vi "数据查询_仪器数据_古田户外.vi"() -> ()   [LabVIEW 2016]
uses:
  <vilib>/Utility/miscctls.llb/LVRowAndColumnUnsignedTypeDef.ctl
  <vilib>/Utility/miscctls.llb/LVPointTypeDef.ctl
panel:
  in  "工作模式":string(combo)="全部数据"
  in  "查询":bool
  in  "结束日期":string="2020/01/01"
  in  "起始日期":string="2010/01/01"
  in  "组合框":string(combo)
  out "数据表":string[][](table)
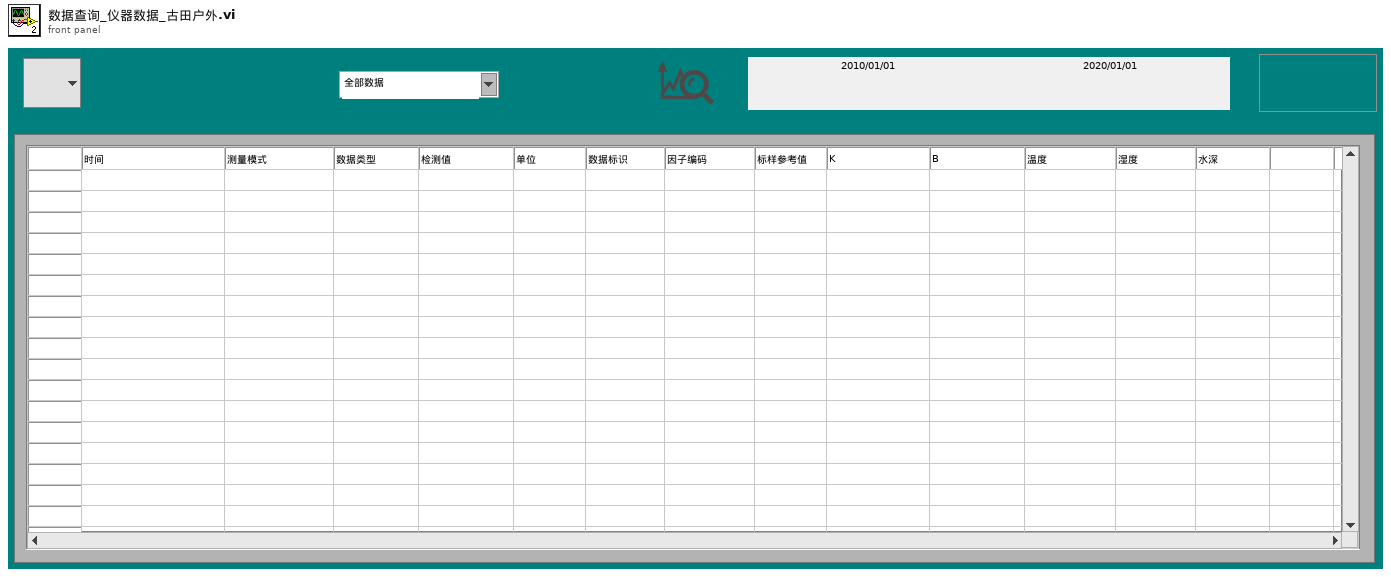
[diagram p1: front panel]
types:
  T1 = typedef "LVRowAndColumnUnsignedTypeDef.ctl" = cluster{"Row":u32, "Column":u32}
  T2 = typedef "LVPointTypeDef.ctl" = cluster{"Horizontal":i16, "Vertical":i16}
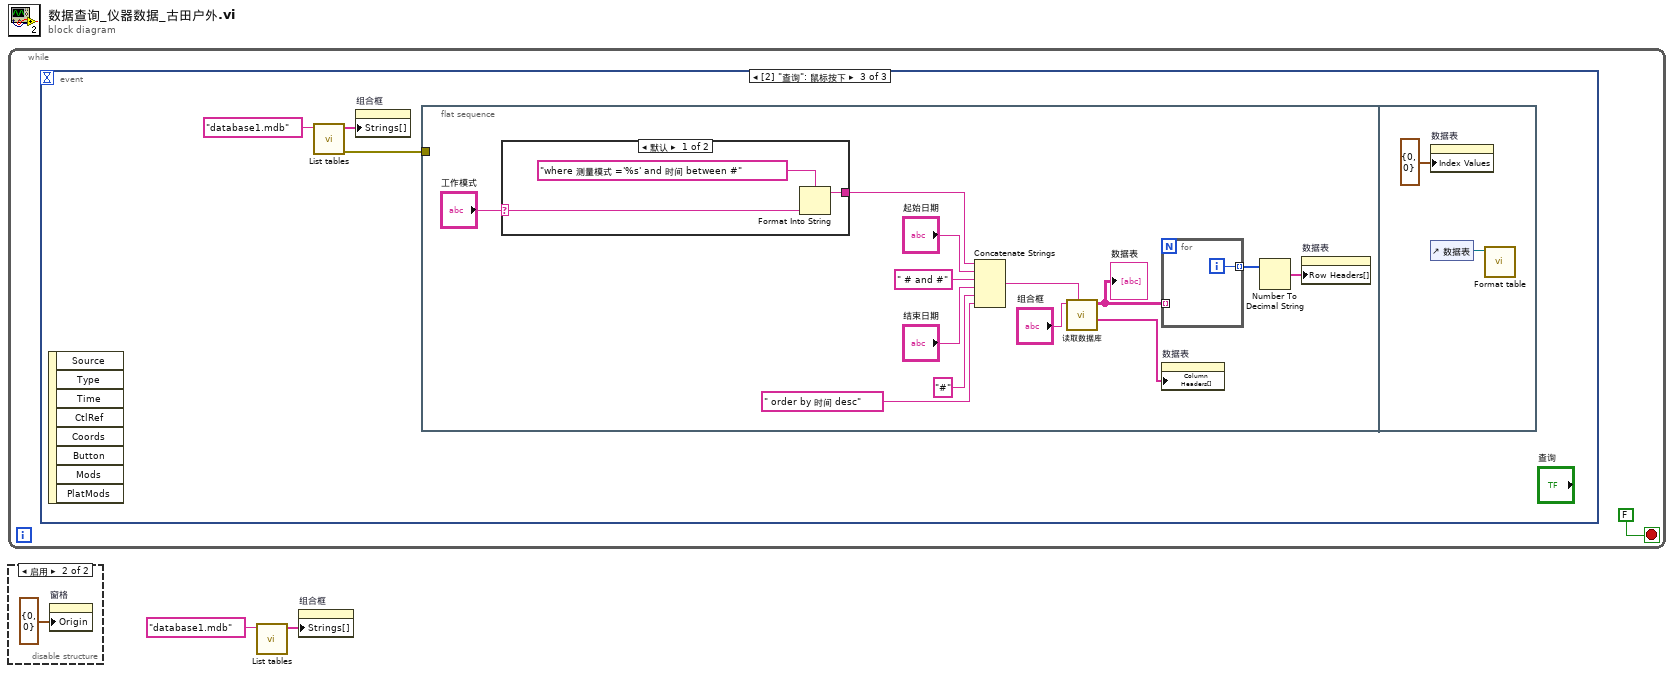
[diagram p0: block diagram]
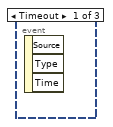
[diagram p2: hidden frame]
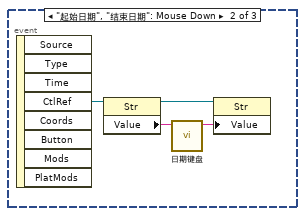
[diagram p3: hidden frame]
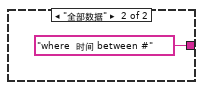
[diagram p4: hidden frame]
diagram:
  n1 = while {
    stop <- FALSE stop-if-true
    n2 = event shown="[2] \"查询\": 鼠标按下" {
      selector: _ -> [_ _ _]
      dyn-events: _ -> [_ _ _]
      timeout: _ -> [_ _ _]
      event Timeout {
        n3 = event-data() -> ()  [unwired: 1 in, 3 out]
      }
      event "起始日期", "结束日期": Mouse Down {
        n4 = event-data() -> ("CtlRef"=w7:refnum<vi>)  [unwired: 1 in, 7 out]
        n5 = property class="Str"(reference=w7) -> (reference out=w5:refnum<vi>, "Value"=w6:string)  [unwired: 1 in, 1 out]
        n6 = call "日期键盘.vi"("原值"=w6) -> ("x+y"=w4:string)  [unwired: 10 in]
        n7 = property class="Str"(reference=w5, "Value"=w4) -> ()  [unwired: 1 in, 2 out]
      }
      event "查询": Mouse Down {
        n8 = event-data() -> ()  [unwired: 1 in, 8 out]
        n9 = call "List tables.vi"("database"="database1.mdb") -> ("error out"=w8:errorcluster, "tables"=w10:string[])  [unwired: 9 in]
        n10 = property on="组合框" class="CmbBox"("Strings[]"=w10) -> ()  [unwired: 2 in, 2 out]
        n11 = flat-sequence {
          tunnel: w8 -> [_]
          frame #0 {
            n12 = case shown="默认" "工作模式" {
              selector: "工作模式" -> [w26 _]
              tunnel: [w24 "where  时间 between #" ("condition")] -> w11
              frame Default {
                n13 = Format Into String(format string="where 测量模式 ='%s' and 时间 between #" ("condition"), w26) -> (resulting string=w24:string)  [unwired: 2 in, 1 out]
              }
              frame "全部数据" {
              }
            }
            n14 = Concatenate Strings(w11, "起始日期", " # and #" ("condition"), "结束日期", "#" ("condition"), " order by 时间 desc" ("字符串")) -> (w22:string)
            n15 = call "读取数据库.vi"("condition"=w22, "组合框"="组合框") -> ("columns"=w18:string[], "表格"=w15:string[][])  [unwired: 6 in, 2 out]
            "数据表" <- w15
            n16 = for {
              tunnel: w15 -> [_] mode=indexing
              tunnel: [w28] -> w14 mode=indexing
              i -> [w28]
            }
            n17 = property on="数据表" class="Tbl (严格)"("Column Headers[]"=w18) -> ()  [unwired: 2 in, 2 out]
            n18 = Number To Decimal String(number=w14) -> (decimal integer string=w13:string[])  [unwired: 1 in]
            n19 = property on="数据表" class="Tbl (严格)"("Row Headers[]"=w13) -> ()  [unwired: 2 in, 2 out]
          }
          frame #1 {
            n20 = property on="数据表" class="Tbl (严格)"("Index Values"=T1 {"Row"=0, "Column"=0} ("索引值")) -> ()  [unwired: 2 in, 2 out]
            n21 = control-ref of="数据表"() -> (w29:refnum<vi>)
            n22 = call "Format table.vi"("Table输入"=w29) -> ()  [unwired: 11 in]
          }
        }
      }
    }
  }
  n23 = disable-structure shown="启用" {
    frame Disabled {
    }
    frame Enabled {
      n24 = property on="窗格" class="Pane"("Origin"=T2 {"Horizontal"=0, "Vertical"=0} ("原点")) -> ()  [unwired: 2 in, 2 out]
    }
  }
  n25 = call "List tables.vi"("database"="database1.mdb") -> ("tables"=w1:string[])  [unwired: 9 in, 1 out]
  n26 = property on="组合框" class="CmbBox"("Strings[]"=w1) -> ()  [unwired: 2 in, 2 out]
